vi "clnt_ck.vi"   [LabVIEW 2012]
uses:
  <vilib>/addons/internet/NI_InternetTK_Core_VIs.lvlib
  <vilib>/addons/internet/NI_InternetTK_Common_VIs.lvlib
types:
  T1 = typedef "CGI Connection Info.ctl" = cluster{"name":string, "type":T2, "session":T3}
  T2 = typedef "CGI Request Type.ctl" = enum16{"cgi", ".spool first", ".spool", ".spool last"}
  T3 = typedef "HTTP Session.ctl" = refnum<k1>
  T4 = typedef "NI_FTP.lvlib/Keyed Array.ctl" = cluster{"keys":string[], "values":string[]}
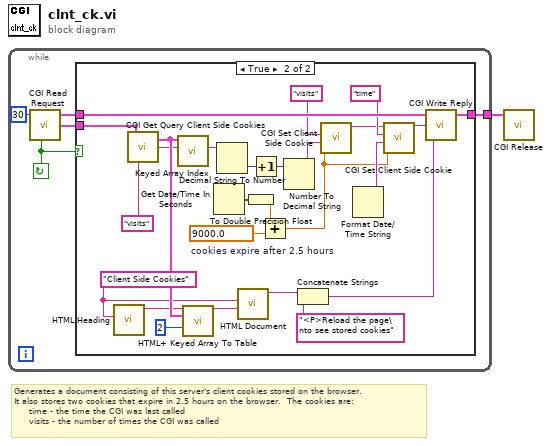
[diagram p0: block diagram]
diagram:
  # "Generates a document consisting of this server's client cookies stored on the browser.\nIt also stores two cookies that expire in 2.5 hours on the browser.  The cookies are:\n     time - the time the CGI was last called\n     visits - the number of times the CGI was called"
  n1 = while {
    tunnel: [w5] -> w1
    stop <- w4 continue-if-true
    n2 = call <vilib>:"CGI Read Request.vi"("timeout in secs (default)"=30) -> ("valid request?"=w4:bool, "cgi connection info"=w6:T1, "env"=w3:T4)  [unwired: 3 in, 1 out]
    n3 = case shown="True" w4 {
      tunnel: [w7 w32] -> w5
      tunnel: w6 -> [w7 w31]
      tunnel: w3 -> [_ w19]
      frame False {
      }
      frame True {
        w22 = 9000.0  # cookies expire after 2.5 hours
        w11 = "Client Side Cookies" ("document title")
        n4 = call <vilib>:"HTML Heading.vi"("heading"=w11) -> ("HTML out"=w12:string)  [unwired: 10 in]
        n5 = call <vilib>:"CGI Get Query Client Side Cookies.vi"("env"=w19) -> ("client cookies"=w18:T4)  [unwired: 1 in, 1 out]
        n6 = call <vilib>:"Keyed Array Index.vi"("key"="visits" ("cookie name"), "array in"=w18) -> ("value"=w16:string)  [unwired: 3 in, 2 out]
        n7 = call <vilib>:"HTML+ Keyed Array To Table.vi"("HTML in"=w12, "keyed array"=w18, "border width (default)"=2) -> ("HTML out"=w29:string)  [unwired: 12 in]
        n8 = Get Date/Time In Seconds() -> (seconds since 1Jan1904=w8:timestamp)
        n9 = Decimal String To Number(string=w16) -> (number=w15:i32)  [unwired: 2 in, 1 out]
        n10 = call <vilib>:"HTML Document.vi"("document body"=w29, "document title"=w11) -> ("HTML Document"=w30:string)  [unwired: 9 in]
        n11 = To Double Precision Float(number=w8) -> (double precision float=w23:dbl)
        n12 = Increment(x=w15) -> (x+1=w14:i32)
        n13 = Add(x=w23, y=w22) -> (x+y=w21:dbl)
        n14 = Number To Decimal String(number=w14) -> (decimal integer string=w13:string)  [unwired: 1 in]
        n15 = Concatenate Strings(w30, "<P>Reload the page\nto see stored cookies") -> (w10:string)
        n16 = call <vilib>:"CGI Set Client Side Cookie.vi"("expires (default)"=w21, "cookie value"=w13, "cookie name"="visits") -> ("header out"=w25:string)  [unwired: 8 in]
        n17 = Format Date/Time String() -> (date/time string=w26:string)  [unwired: 3 in]
        n18 = call <vilib>:"CGI Set Client Side Cookie.vi"("expires (default)"=w21, "cookie value"=w26, "cookie name"="time", "header in"=w25) -> ("header out"=w28:string)  [unwired: 7 in]
        n19 = call <vilib>:"CGI Write Reply.vi"("content"=w10, "header"=w28, "cgi connection info"=w31) -> ("cgi connection info out"=w32:T1)  [unwired: 2 in]
      }
    }
  }
  n20 = call <vilib>:"CGI Release.vi"("cgi connection info"=w1) -> ()  [unwired: 5 in]
